vi "PC104_interface.vi"() -> ()   [LabVIEW 2016]
uses:
  <vilib>/httpClient/LabVIEWHTTPClient.lvlib
  <vilib>/httpClient/ClientHandle.ctl
  <vilib>/httpClient/POSTBuffer.vi
  msg7171_linux.llb/send single message.vi
  Type_Defs/Digital_Out.ctl
  Type_Defs/Digital_In_1.ctl
  Type_Defs/Analog_In.ctl
panel:
  in  "IR Lamps DutyCycle":dbl[][](array[numeric])
  out "Analog in":T1
  in  "LN2 Platen":u16(slide) max=4095 step=1 scale=0.0..4095.0
  in  "LN2 Shroud":u16(slide) max=4095 step=1 scale=0.0..4095.0
  out "Digi_In_1":T2
  in  "Digi_Out":T3
  in  "Get DIO":bool=TRUE
  in  "exit":bool
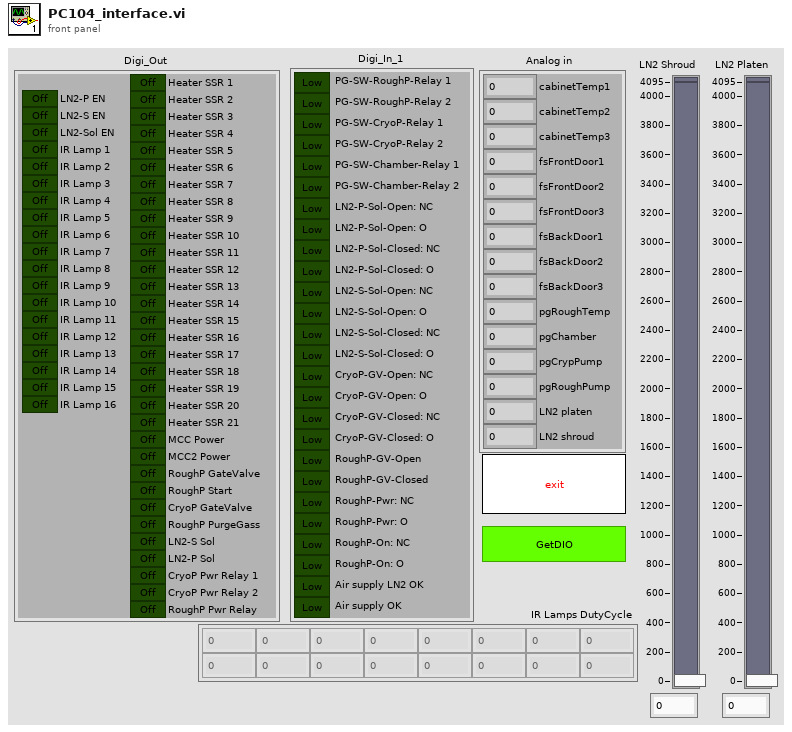
[diagram p1: front panel]
types:
  T1 = typedef "Analog_In.ctl" = cluster{"cabinetTemp1":u16, "cabinetTemp2":u16, "cabinetTemp3":u16, "fsFrontDoor1":u16, "fsFrontDoor2":u16, "fsFrontDoor3":u16, "fsBackDoor1":u16, "fsBackDoor2":u16, "fsBackDoor3":u16, "pgRoughTemp":u16, "pgChamber":u16, "pgCrypPump":u16, "pgRoughPump":u16, "LN2 platen":u16, "LN2 shroud":u16}
  T2 = typedef "Digital_In_1.ctl" = cluster{"PG-SW-RoughP-Relay 1":bool, "PG-SW-RoughP-Relay 2":bool, "PG-SW-CryoP-Relay 1":bool, "PG-SW-CryoP-Relay 2":bool, "PG-SW-Chamber-Relay 1":bool, "PG-SW-Chamber-Relay 2":bool, "LN2-P-Sol-Open: NC":bool, "LN2-P-Sol-Open: O":bool, "LN2-P-Sol-Closed: NC":bool, "LN2-P-Sol-Closed: O":bool, "LN2-S-Sol-Open: NC":bool, "LN2-S-Sol-Open: O":bool, "LN2-S-Sol-Closed: NC":bool, "LN2-S-Sol-Closed: O":bool, "CryoP-GV-Open: NC":bool, "CryoP-GV-Open: O":bool, "CryoP-GV-Closed: NC":bool, "CryoP-GV-Closed: O":bool, "RoughP-GV-Open":bool, "RoughP-GV-Closed":bool, "RoughP-Pwr: NC":bool, "RoughP-Pwr: O":bool, "RoughP-On: NC":bool, "RoughP-On: O":bool, "Air supply LN2 OK":bool, "Air supply OK":bool}
  T3 = typedef "Digital_Out.ctl" = cluster{"LN2-P EN":bool, "LN2-S EN":bool, "LN2-Sol EN":bool, "IR Lamp 1":bool, "IR Lamp 2":bool, "IR Lamp 3":bool, "IR Lamp 4":bool, "IR Lamp 5":bool, "IR Lamp 6":bool, "IR Lamp 7":bool, "IR Lamp 8":bool, "IR Lamp 9":bool, "IR Lamp 10":bool, "IR Lamp 11":bool, "IR Lamp 12":bool, "IR Lamp 13":bool, "IR Lamp 14":bool, "IR Lamp 15":bool, "IR Lamp 16":bool, "Heater SSR 1":bool, "Heater SSR 2":bool, "Heater SSR 3":bool, "Heater SSR 4":bool, "Heater SSR 5":bool, "Heater SSR 6":bool, "Heater SSR 7":bool, "Heater SSR 8":bool, "Heater SSR 9":bool, "Heater SSR 10":bool, "Heater SSR 11":bool, "Heater SSR 12":bool, "Heater SSR 13":bool, "Heater SSR 14":bool, "Heater SSR 15":bool, "Heater SSR 16":bool, "Heater SSR 17":bool, "Heater SSR 18":bool, "Heater SSR 19":bool, "Heater SSR 20":bool, "Heater SSR 21":bool, "MCC Power":bool, "MCC2 Power":bool, "RoughP GateValve":bool, "RoughP Start":bool, "CryoP GateValve":bool, "RoughP PurgeGass":bool, "LN2-S Sol":bool, "LN2-P Sol":bool, "CryoP Pwr Relay 1":bool, "CryoP Pwr Relay 2":bool, "RoughP Pwr Relay":bool}
  T4 = typedef "LabVIEWHTTPClient.lvlib/ClientHandle.ctl" = refnum<k1>
  T5 = cluster{"go":bool, "Http session":T4, "URL prefex":string}
  T6 = cluster{"out":cluster{"LN2 Platen":u16, "LN2 Shroud":u16}, "in":T1}
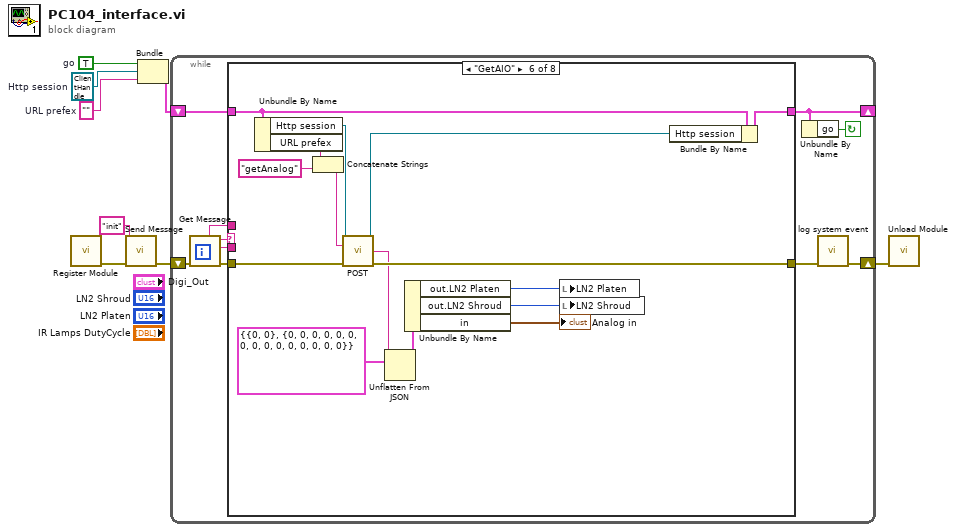
[diagram p0: block diagram]
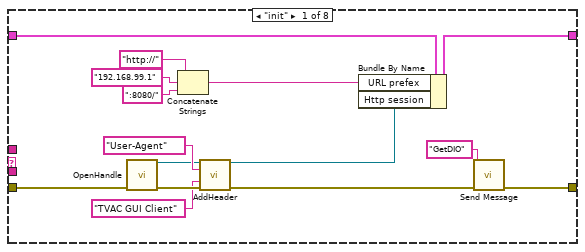
[diagram p2: hidden frame]
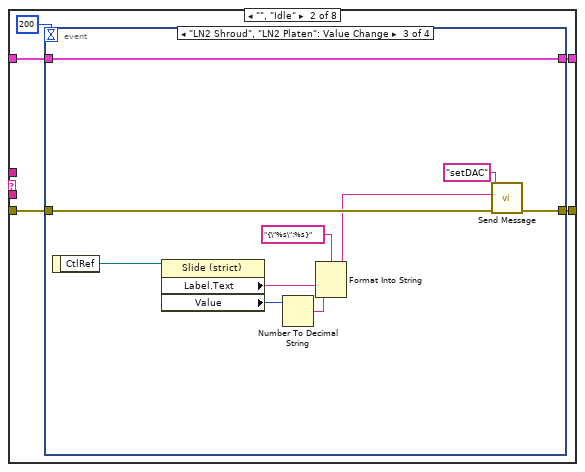
[diagram p3: hidden frame]
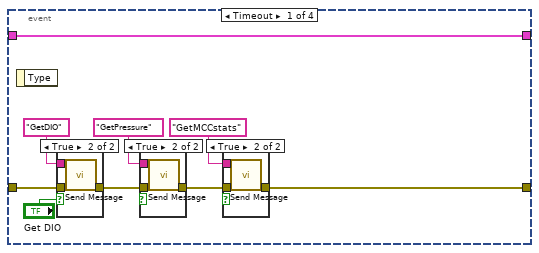
[diagram p4: hidden frame]
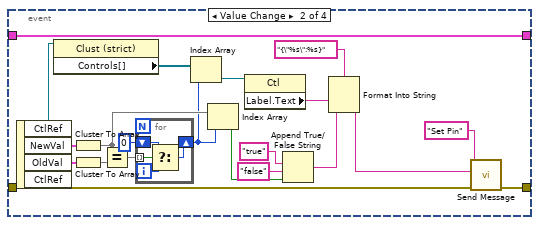
[diagram p8: hidden frame]
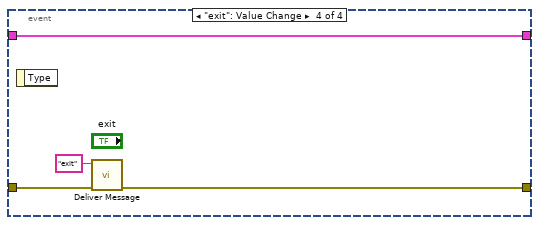
[diagram p9: hidden frame]
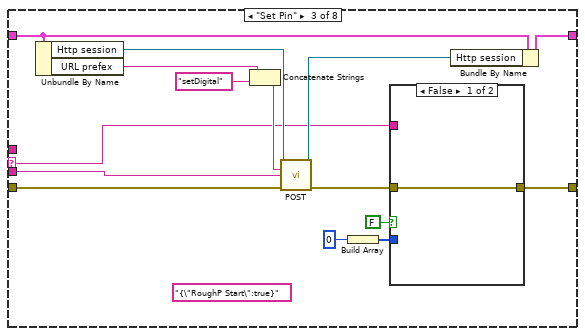
[diagram p10: hidden frame]
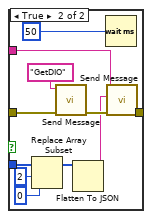
[diagram p11: hidden frame]
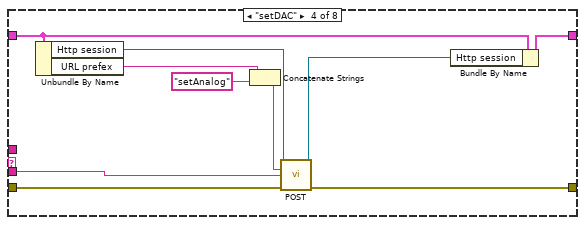
[diagram p12: hidden frame]
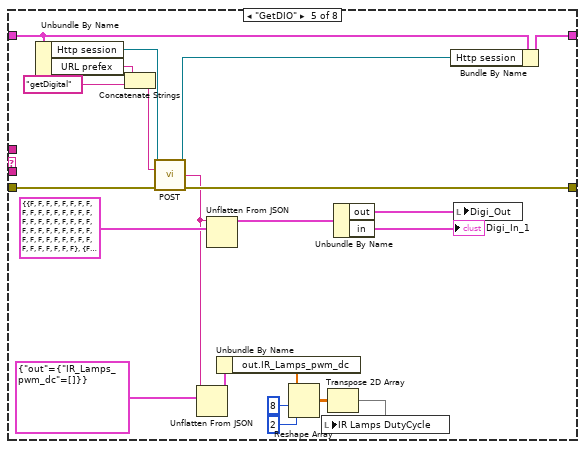
[diagram p13: hidden frame]
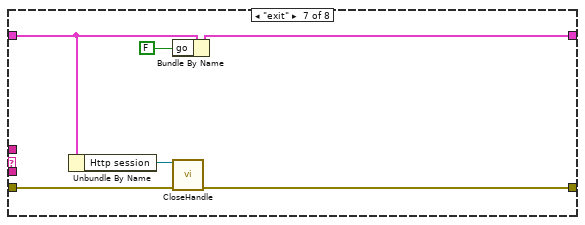
[diagram p14: hidden frame]
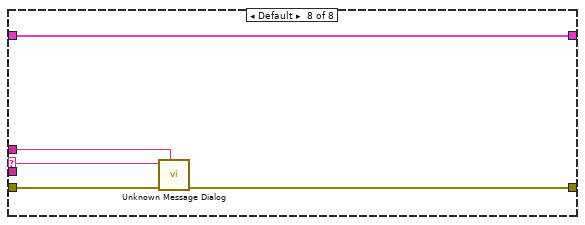
[diagram p15: hidden frame]
diagram:
  w4 = ""  # URL prefex
  w5 = T4 refnum  # Http session
  w6 = TRUE  # go
  n1 = call "Register Module.vi"() -> ("error out"=w2:errorcluster)  [unwired: 10 in, 1 out]
  n2 = call-poly "Send Message.vi"("error in (no error)"=w2, "event"="init") -> ("error out"=w1:errorcluster)  [unwired: 9 in]
  n3 = Bundle("go"=w6, "Http session"=w5, "URL prefex"=w4) -> (w8:T5)  [unwired: 1 in]
  n4 = while {
    shift-left: w8 -> [w15]
    shift-right: [w12] -> _
    shift-right: [w10] -> w7
    shift-left: w1 -> [w18]
    stop <- w11 continue-if-true
    n5 = call "Get Message.vi"("error in (no error)"=w18) -> ("error out"=w16:errorcluster, "event buffer"=w17:string, "event"=w14:string, "source"=w13:string)  [unwired: 7 in]
    n6 = case shown="\"GetAIO\"" w14 {
      selector: w14 -> [_ _ w104 _ _ _ _ w180]
      tunnel: [w24 w35 w108 w130 w149 w164 w177 w182] -> w12
      tunnel: w15 -> [w33 w34 w107 w129 w148 w163 w172 w182]
      tunnel: w17 -> [_ _ w102 w126 _ _ _ _]
      tunnel: w16 -> [w28 w36 w106 w128 w151 w166 w175 w181]
      tunnel: w13 -> [_ _ _ _ _ _ _ w179]
      tunnel: [w20 w38 w105 w127 w150 w165 w174 w178] -> w9
      frame "init" {
        n7 = call <vilib>:"OpenHandle.vi"("error in (no error)"=w28) -> ("client handle out"=w29:T4, "error out"=w32:errorcluster)  [unwired: 13 in]
        n8 = Concatenate Strings("http://" ("url"), "192.168.99.1" ("Address"), ":8080/" ("url")) -> (w23:string)
        n9 = call <vilib>:"AddHeader.vi"("client handle"=w29, "header"="User-Agent", "value"="TVAC GUI Client", "error in (no error)"=w32) -> ("client handle out"=w22:T4, "error out"=w21:errorcluster)  [unwired: 10 in]
        n10 = Bundle By Name(cluster=w33, "URL prefex"=w23, "Http session"=w22) -> (w24:T5)
        n11 = call-poly "Send Message.vi"("error in (no error)"=w21, "event"="GetDIO") -> ("error out"=w20:errorcluster)  [unwired: 9 in]
      }
      frame "", "Idle" {
        n12 = event shown="[2] \"LN2 Shroud\", \"LN2 Platen\": Value Change" {
          selector: _ -> [_ _ _ _]
          dyn-events: _ -> [_ _ _ _]
          timeout: 200 ("milliseconds to wait") -> [_ _ _ _]
          tunnel: w36 -> [w46 w75 w92 w98]
          tunnel: [w39 w74 w93 w97] -> w38
          tunnel: [w47 w80 w85 w95] -> w35
          tunnel: w34 -> [w47 w80 w85 w95]
          event Timeout {
            n13 = event-data() -> ()  [unwired: 1 in, 1 out]
            n14 = case shown="True" "Get DIO" {
              tunnel: w46 -> [w56 w59]
              tunnel: [w56 w58] -> w44
              tunnel: "GetDIO" ("event") -> [_ w57]
              frame False {
              }
              frame True {
                n15 = call-poly "Send Message.vi"("error in (no error)"=w59, "event"=w57) -> ("error out"=w58:errorcluster)  [unwired: 9 in]
              }
            }
            n16 = case shown="True" {
              selector: _ -> [_ _]
              tunnel: w44 -> [w52 w55]
              tunnel: [w52 w54] -> w40
              tunnel: "GetPressure" ("event") -> [_ w53]
              frame False {
              }
              frame True {
                n17 = call-poly "Send Message.vi"("error in (no error)"=w55, "event"=w53) -> ("error out"=w54:errorcluster)  [unwired: 9 in]
              }
            }
            n18 = case shown="True" {
              selector: _ -> [_ _]
              tunnel: w40 -> [w48 w51]
              tunnel: [w48 w50] -> w39
              tunnel: "GetMCCstats" ("event") -> [_ w49]
              frame False {
              }
              frame True {
                n19 = call-poly "Send Message.vi"("error in (no error)"=w51, "event"=w49) -> ("error out"=w50:errorcluster)  [unwired: 9 in]
              }
            }
          }
          event Value Change {
            n20 = event-data() -> ("CtlRef"=w61:refnum<vi>, "NewVal"=w76:T3, "OldVal"=w79:T3)  [unwired: 1 in, 1 out]
            n21 = property class="Clust (strict)"(reference=w61) -> ("Controls[]"=w71:refnum<vi>[])  [unwired: 1 in, 2 out]
            n22 = Cluster To Array(cluster=w76) -> (array=w72:bool[])
            n23 = Cluster To Array(cluster=w79) -> (array=w73:bool[])
            n24 = Equal?(x=w72, y=w73) -> (x = y?=w78:bool[])
            n25 = for {
              tunnel: w78 -> [w84] mode=indexing
              shift-right: [w83] -> w70
              shift-left: 0 -> [w82]
              i -> [w81]
              n26 = Select(t=w82, s=w84, f=w81) -> (s? t:f=w83:i32)
            }
            n27 = Index Array(array=w71, index=w70) -> (element=w69:refnum<vi>)
            n28 = Index Array(array=w72, index=w70) -> (element=w67:bool)
            n29 = property class="Ctl"(reference=w69) -> ("Label.Text"=w64:string)  [unwired: 1 in, 2 out]
            n30 = Append True/False String(1:w67, 2:"false" ("false string"), 3:"true" ("true string")) -> (0:w62:string)  [unwired: 1 in]
            n31 = Format Into String(format string="{\"%s\":%s}" ("string"), w64, w62) -> (resulting string=w60:string)  [unwired: 2 in, 1 out]
            n32 = call-poly "Send Message.vi"("error in (no error)"=w75, "event buffer"=w60, "event"="Set Pin") -> ("error out"=w74:errorcluster)  [unwired: 8 in]
          }
          event "LN2 Shroud", "LN2 Platen": Value Change {
            n33 = event-data() -> ("CtlRef"=w91:refnum<vi>)  [unwired: 1 in]
            n34 = property class="Slide (strict)"(reference=w91) -> ("Label.Text"=w89:string, "Value"=w88:u16)  [unwired: 1 in, 2 out]
            n35 = Number To Decimal String(number=w88) -> (decimal integer string=w87:string)  [unwired: 1 in]
            n36 = Format Into String(format string="{\"%s\":%s}" ("string"), w89, w87) -> (resulting string=w86:string)  [unwired: 2 in, 1 out]
            n37 = call-poly "Send Message.vi"("error in (no error)"=w92, "event buffer"=w86, "event"="setDAC") -> ("error out"=w93:errorcluster)  [unwired: 8 in]
          }
          event "exit": Value Change {
            n38 = event-data() -> ()  [unwired: 1 in, 1 out]
            n39 = call "Deliver Message.vi"("error in (no error)"=w98, "event"="exit") -> ("error out"=w97:errorcluster)  [unwired: 9 in]
          }
        }
      }
      frame "Set Pin" {
        (unwired) "{\"RoughP Start\":true}" ("string")
        n40 = Unbundle By Name(w107) -> ("Http session"=w112:T4, "URL prefex"=w110:string)
        n41 = Concatenate Strings(w110, "setDigital" ("url")) -> (w111:string)
        n42 = call-poly <vilib>:"POST.vi"("client handle"=w112, "url"=w111, "buffer"=w102, "error in (no error)"=w106) -> ("client handle out"=w113:T4, "error out"=w103:errorcluster)  [unwired: 8 in, 2 out]
        n43 = Build Array(0) -> (w100:i32[])
        n44 = case shown="False" FALSE {
          tunnel: [w114 w125] -> w105
          tunnel: w104 -> [_ w124]
          tunnel: w103 -> [w114 w123]
          tunnel: w100 -> [_ w120]
          frame False {
          }
          frame True {
            n45 = Replace Array Subset(array=w120, new element=0 ("new element/subarray"), index=2) -> (w116:i32[])
            n46 = call-poly "Send Message.vi"("error in (no error)"=w123, "event"="GetDIO") -> ("error out"=w122:errorcluster)  [unwired: 9 in]
            n47 = Flatten To JSON(anything=w116) -> (JSON string=w117:string)  [unwired: 2 in, 1 out]
            n48 = Wait (ms)(milliseconds to wait=u32 50) -> ()  [unwired: 1 out]
            n49 = call-poly "Send Message.vi"("error in (no error)"=w122, "event buffer"=w117, "event"=w124) -> ("error out"=w125:errorcluster)  [unwired: 8 in]
          }
        }
        n50 = Bundle By Name(cluster=w107, "Http session"=w113) -> (w108:T5)
      }
      frame "setDAC" {
        n51 = Unbundle By Name(w129) -> ("Http session"=w134:T4, "URL prefex"=w132:string)
        n52 = Concatenate Strings(w132, "setAnalog" ("url")) -> (w133:string)
        n53 = call-poly <vilib>:"POST.vi"("client handle"=w134, "url"=w133, "buffer"=w126, "error in (no error)"=w128) -> ("client handle out"=w135:T4, "error out"=w127:errorcluster)  [unwired: 8 in, 2 out]
        n54 = Bundle By Name(cluster=w129, "Http session"=w135) -> (w130:T5)
      }
      frame "GetDIO" {
        n55 = Unbundle By Name(w148) -> ("Http session"=w155:T4, "URL prefex"=w153:string)
        n56 = Concatenate Strings(w153, "getDigital" ("url")) -> (w154:string)
        n57 = call-poly <vilib>:"POST.vi"("client handle"=w155, "url"=w154, "error in (no error)"=w151) -> ("client handle out"=w156:T4, "body"=w136:string, "error out"=w150:errorcluster)  [unwired: 9 in, 1 out]
        n58 = Unflatten From JSON(JSON string=w136, type and defaults=cluster{"out":cluster{"IR_Lamps_pwm_dc":dbl[]}} {"out"={"IR_Lamps_pwm_dc"=[]}}) -> (value=w138:cluster{"out":cluster{"IR_Lamps_pwm_dc":dbl[]}})  [unwired: 5 in, 1 out]
        n59 = Unflatten From JSON(JSON string=w136, type and defaults=cluster{"out":T3, "in":T2} {"out"={"LN2-P EN"=FALSE, "LN2-S EN"=FALSE, "LN2-Sol EN"=FALSE, "IR Lamp 1"=FALSE, "IR Lamp 2"=FALSE, "IR Lamp 3"=FALSE, "IR Lamp 4"=FALSE, "IR Lamp 5"=FALSE, "IR Lamp 6"=FALSE, "IR Lamp 7"=FALSE, "IR Lamp 8"=FALSE, "IR Lamp 9"=FALSE, "IR Lamp 10"=FALSE, "IR Lamp 11"=FALSE, "IR Lamp 12"=FALSE, "IR Lamp 13"=FALSE, "IR Lamp 14"=FALSE, "IR Lamp 15"=FALSE, "IR Lamp 16"=FALSE, "Heater SSR 1"=FALSE, "Heater SSR 2"=FALSE, "Heater SSR 3"=FALSE, "Heater SSR 4"=FALSE, "Heater SSR 5"=FALSE, "Heater SSR 6"=FALSE, "Heater SSR 7"=FALSE, "Heater SSR 8"=FALSE, "Heater SSR 9"=FALSE, "Heater SSR 10"=FALSE, "Heater SSR 11"=FALSE, "Heater SSR 12"=FALSE, "Heater SSR 13"=FALSE, "Heater SSR 14"=FALSE, "Heater SSR 15"=FALSE, "Heater SSR 16"=FALSE, "Heater SSR 17"=FALSE, "Heater SSR 18"=FALSE, "Heater SSR 19"=FALSE, "Heater SSR 20"=FALSE, "Heater SSR 21"=FALSE, "MCC Power"=FALSE, "MCC2 Power"=FALSE, "RoughP GateValve"=FALSE, "RoughP Start"=FALSE, "CryoP GateValve"=FALSE, "RoughP PurgeGass"=FALSE, "LN2-S Sol"=FALSE, "LN2-P Sol"=FALSE, "CryoP Pwr Relay 1"=FALSE, "CryoP Pwr Relay 2"=FALSE, "RoughP Pwr Relay"=FALSE}, "in"={"PG-SW-RoughP-Relay 1"=FALSE, "PG-SW-RoughP-Relay 2"=FALSE, "PG-SW-CryoP-Relay 1"=FALSE, "PG-SW-CryoP-Relay 2"=FALSE, "PG-SW-Chamber-Relay 1"=FALSE, "PG-SW-Chamber-Relay 2"=FALSE, "LN2-P-Sol-Open: NC"=FALSE, "LN2-P-Sol-Open: O"=FALSE, "LN2-P-Sol-Closed: NC"=FALSE, "LN2-P-Sol-Closed: O"=FALSE, "LN2-S-Sol-Open: NC"=FALSE, "LN2-S-Sol-Open: O"=FALSE, "LN2-S-Sol-Closed: NC"=FALSE, "LN2-S-Sol-Closed: O"=FALSE, "CryoP-GV-Open: NC"=FALSE, "CryoP-GV-Open: O"=FALSE, "CryoP-GV-Closed: NC"=FALSE, "CryoP-GV-Closed: O"=FALSE, "RoughP-GV-Open"=FALSE, "RoughP-GV-Closed"=FALSE, "RoughP-Pwr: NC"=FALSE, "RoughP-Pwr: O"=FALSE, "RoughP-On: NC"=FALSE, "RoughP-On: O"=FALSE, "Air supply LN2 OK"=FALSE, "Air supply OK"=FALSE}}) -> (value=w144:cluster{"out":T3, "in":T2})  [unwired: 5 in, 1 out]
        n60 = Unbundle By Name(w138) -> ("out.IR_Lamps_pwm_dc"=w137:dbl[])
        n61 = Reshape Array(w137, 8 ("dimension size"), 2 ("dimension size")) -> (w141:dbl[][])
        n62 = Transpose 2D Array(2D array=w141) -> (transposed array=w140:dbl[][])
        n63 = local write "IR Lamps DutyCycle"(w140) -> ()
        n64 = Unbundle By Name(w144) -> ("out"=w147:T3, "in"=→"Digi_In_1":T2)
        n65 = Bundle By Name(cluster=w148, "Http session"=w156) -> (w149:T5)
        n66 = local write "Digi_Out"(w147) -> ()
      }
      frame "GetAIO" {
        n67 = Unbundle By Name(w163) -> ("Http session"=w170:T4, "URL prefex"=w168:string)
        n68 = Concatenate Strings(w168, "getAnalog" ("url")) -> (w169:string)
        n69 = call-poly <vilib>:"POST.vi"("client handle"=w170, "url"=w169, "error in (no error)"=w166) -> ("client handle out"=w171:T4, "body"=w160:string, "error out"=w165:errorcluster)  [unwired: 9 in, 1 out]
        n70 = Unflatten From JSON(JSON string=w160, type and defaults=T6 {"out"={"LN2 Platen"=0, "LN2 Shroud"=0}, "in"={"cabinetTemp1"=0, "cabinetTemp2"=0, "cabinetTemp3"=0, "fsFrontDoor1"=0, "fsFrontDoor2"=0, "fsFrontDoor3"=0, "fsBackDoor1"=0, "fsBackDoor2"=0, "fsBackDoor3"=0, "pgRoughTemp"=0, "pgChamber"=0, "pgCrypPump"=0, "pgRoughPump"=0, "LN2 platen"=0, "LN2 shroud"=0}}) -> (value=w161:T6)  [unwired: 5 in, 1 out]
        n71 = Unbundle By Name(w161) -> ("out.LN2 Platen"=w158:u16, "out.LN2 Shroud"=w157:u16, "in"=→"Analog in":T1)
        n72 = local write "LN2 Platen"(w158) -> ()
        n73 = local write "LN2 Shroud"(w157) -> ()
        n74 = Bundle By Name(cluster=w163, "Http session"=w171) -> (w164:T5)
      }
      frame "exit" {
        n75 = Unbundle By Name(w172) -> ("Http session"=w173:T4)
        n76 = Bundle By Name(cluster=w172, "go"=FALSE ("Bundle Element")) -> (w177:T5)
        n77 = call <vilib>:"CloseHandle.vi"("client handle"=w173, "error in (no error)"=w175) -> ("error out"=w174:errorcluster)  [unwired: 13 in]
      }
      frame Default {
        n78 = call "Unknown Message Dialog.vi"("source"=w179, "error in (no error)"=w181, "event name"=w180) -> ("error out"=w178:errorcluster)  [unwired: 8 in]
      }
    }
    n79 = Unbundle By Name(w12) -> ("go"=w11:bool)
    n80 = call "log system event.vi"("error in (no error)"=w9) -> ("error out"=w10:errorcluster)  [unwired: 9 in, 1 out]
  }
  n81 = call "Unload Module.vi"("error in (no error)"=w7) -> ()  [unwired: 10 in, 1 out]
